vi "HandleGameOver.vi"(8 "error in (no error)":errorcluster, 11 "Game in":refnum<class "Game.lvclass">) -> (0 "error out":errorcluster, 3 "Game out":refnum<class "Game.lvclass">)   [LabVIEW 2019, in "RT_Game.lvlib" / "Game.lvclass"]
uses:
  Game.lvclass
  Game.lvclass/Game.ctl
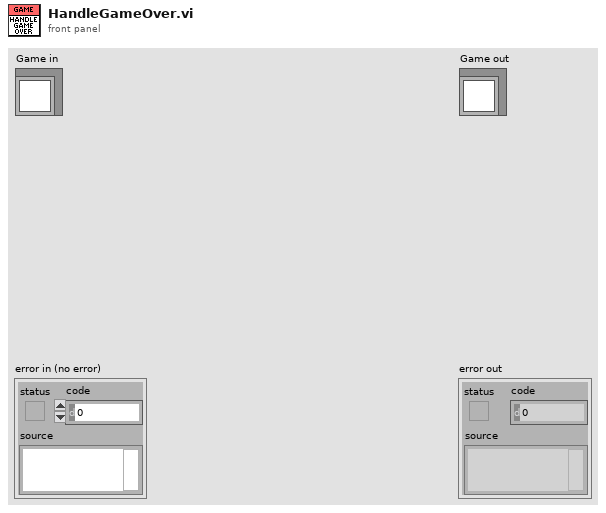
[diagram p1: front panel]
types:
  T1 = typedef "RT_Game.lvlib/Game.lvclass/States.ctl" = enum16{"Init", "Restart", "Menu", "Game", "Resume", "ToggleSingleplayer", "LoadNextGame", "ExitToMenu", "SlideOut"}
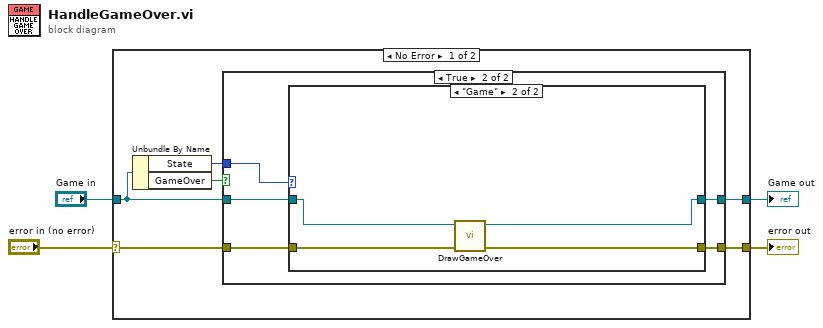
[diagram p0: block diagram]
diagram:
  n1 = case shown="No Error" "error in (no error)" {
    selector: "error in (no error)" -> [w10 w25]
    tunnel: [w9 w25] -> w3
    tunnel: [w8 w24] -> w1
    tunnel: "Game in" -> [w7 w24]
    frame No Error {
      n2 = Unbundle By Name(w7) -> ("State"=w5:T1, "GameOver"=w6:bool)
      n3 = case shown="True" w6 {
        tunnel: w10 -> [w12 w17]
        tunnel: w7 -> [w11 w16]
        tunnel: [w12 w15] -> w9
        tunnel: [w11 w14] -> w8
        tunnel: w5 -> [_ w13]
        frame False {
        }
        frame True {
          n4 = case shown="\"Game\"" w13 {
            tunnel: w17 -> [w18 w23]
            tunnel: w16 -> [w19 w22]
            tunnel: [w18 w21] -> w15
            tunnel: [w19 w20] -> w14
            frame Default {
            }
            frame "Game" {
              n5 = call "DrawGameOver.vi"("error in (no error)"=w23, "Game in"=w22) -> ("error out"=w21:errorcluster, "Game out"=w20:refnum<class "Game.lvclass">)  [unwired: 8 in]
            }
          }
        }
      }
    }
    frame Error {
    }
  }
  "error out" <- w3
  "Game out" <- w1
